vi "Write Reporters.vi"(8 "error in":errorcluster, 10 "Reporters":refnum<class "Reporter.lvclass">[](array[class]), 11 "Report With First Working in":refnum<class "Report With First Working.lvclass">) -> (0 "error out":errorcluster, 3 "Report With First Working out":refnum<class "Report With First Working.lvclass">)   [LabVIEW 2020, in "Approval Tests.lvlib" / "Report With First Working.lvclass"]
uses:
  Report With First Working.lvclass
  Reporter/Reporter.lvclass
  Report With First Working.lvclass/Report With First Working.ctl
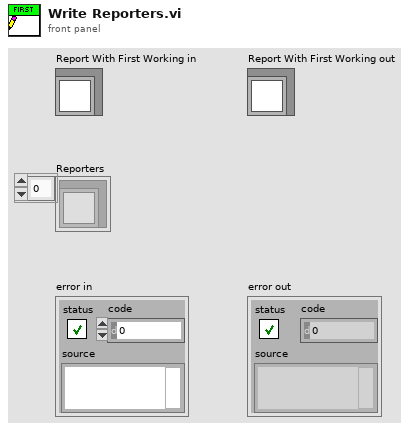
[diagram p1: front panel]
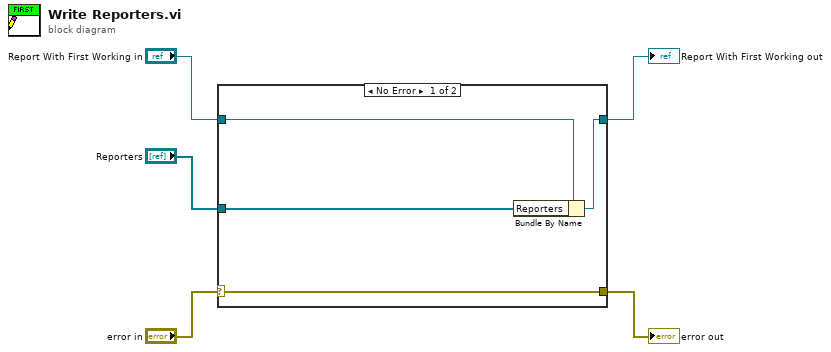
[diagram p0: block diagram]
diagram:
  n1 = case shown="No Error" "error in" {
    selector: "error in" -> [w9 w11]
    tunnel: [w9 w11] -> w4
    tunnel: [w7 w10] -> w2
    tunnel: "Report With First Working in" -> [w8 w10]
    tunnel: "Reporters" -> [w6 _]
    frame No Error {
      n2 = Bundle By Name(cluster=w8, "Reporters"=w6) -> (w7:refnum<class "Report With First Working.lvclass">)
    }
    frame Error {
    }
  }
  "error out" <- w4
  "Report With First Working out" <- w2
